vi "Pick and Place Camera.vi"(0 "Gantry In":refnum<k24>, 1 "XYZTheta":dbl[](array[numeric]), 4 "Position":i32, 5 "Tray Number":i32) -> (7 "Gantry Out":refnum<k24>)   [LabVIEW 2021, in "Pick and Place.lvclass"]
uses:
  Pick and Place.lvclass
  Controller/Camera/Image processing.ctl
  Controller/Camera/Camera settings.ctl
  Workspace/Component/Find Component.ctl
  Controller/Camera/Machine Vision.ctl
  C:/Program Files (x86)/Aerotech/A3200/LabVIEW/2010/Bin/Aerotech.A3200.dll
  Program Files (x86)/Aerotech/A3200/LabVIEW/2010/Bin/Aerotech.A3200.dll
  Controller/Camera/Edmund Optics/Edmund Optics.lvclass
  C:/Users/HEP/Documents/GitHub/Gantry/UCSB-Gantry-HEP-main/Classes/Controller/Camera/Camera.lvclass
  Controller/Camera/Camera.lvclass
  Controller/Motion/A3200/A3200.lvclass
  Controller/Motion/Motion.lvclass
  Workspace/Component/Component Tray.lvclass
panel:
  in  "Machine Vision":T1
  in  "Assembly Type":string
  in  "Component":T2
  in  "Verify CH1":bool
  out "CH1 correct?":bool
  in  "Go to Sensor ID":bool
  in  "Go to CH1":bool
  in  "Go to Center":bool
  in  "Joystick":bool
  in  "Focus":bool
  in  "number of focus steps":i32
  in  "Focus step size":dbl format="%#_13g"
  out "XYZTheta 2":dbl[](array[numeric]) format="%.6g"
  out "All fiducials recorded":bool
  out "CH1 Location":dbl[](array[numeric])
  out "Sensor ID Location":dbl[](array[numeric])
  out "XY Graph":cluster{"X":dbl, "Y":dbl}[](graph)
  out "Bottom Left XY":dbl[](array[numeric]) format="%.6g"
  out "Bottom Right XY":dbl[](array[numeric]) format="%.6g"
  out "Top Right XY":dbl[](array[numeric]) format="%.6g"
  out "Top Left XY":dbl[](array[numeric]) format="%.6g"
  in  "Record Top Left":bool
  in  "Record Top Right":bool
  in  "Record Bottom Right":bool
  in  "Record Bottom Left":bool
  in  "Go to Top Left":bool
  in  "Go to Bottom Left":bool
  in  "Go to Bottom Right":bool
  in  "Go to Top Right":bool
  out "Gantry":dbl[](array[numeric]) format="%.6g"
  out "Sum":dbl[](array[numeric]) format="%.6g"
  out "Low Speed":bool
  out "X":bool
  out "Y":bool
  out "Z":bool
  out "High Speed":bool
  in  "Stop Program":bool
  out "Image":T3(plugin-control)
  out "Camera":dbl[](array[numeric]) format="%.6g"
  in  "Override presets":bool
  in  "Camera settings":T4={"Gamma"=1.6, "Gain"=0, "Sharpness"=0, "Contrast"=0.0, "Exposure"=0.0078125} {"Exposure" min=0.000244140625 max=0.5 scale=0.0002..0.5; "Contrast" min=0.0 max=1.0 scale=0.001..1.0; "Sharpness" min=0 max=2 step=1 scale=0.0..2.0; "Gain" min=0 max=100 step=1 scale=0.1..100.0; "Gamma" min=0.01 max=10.0 scale=0.01..10.0}
  in  "Image processing":T5={"Brightness"=128.0, "Contrast"=45.0, "Gamma"=1.0471123} {"Brightness" scale=0.0..400.0; "Contrast" scale=0.0..90.0; "Gamma" scale=0.005..5.0}
  out "Average Strength":dbl
  out "Program Stopped":bool
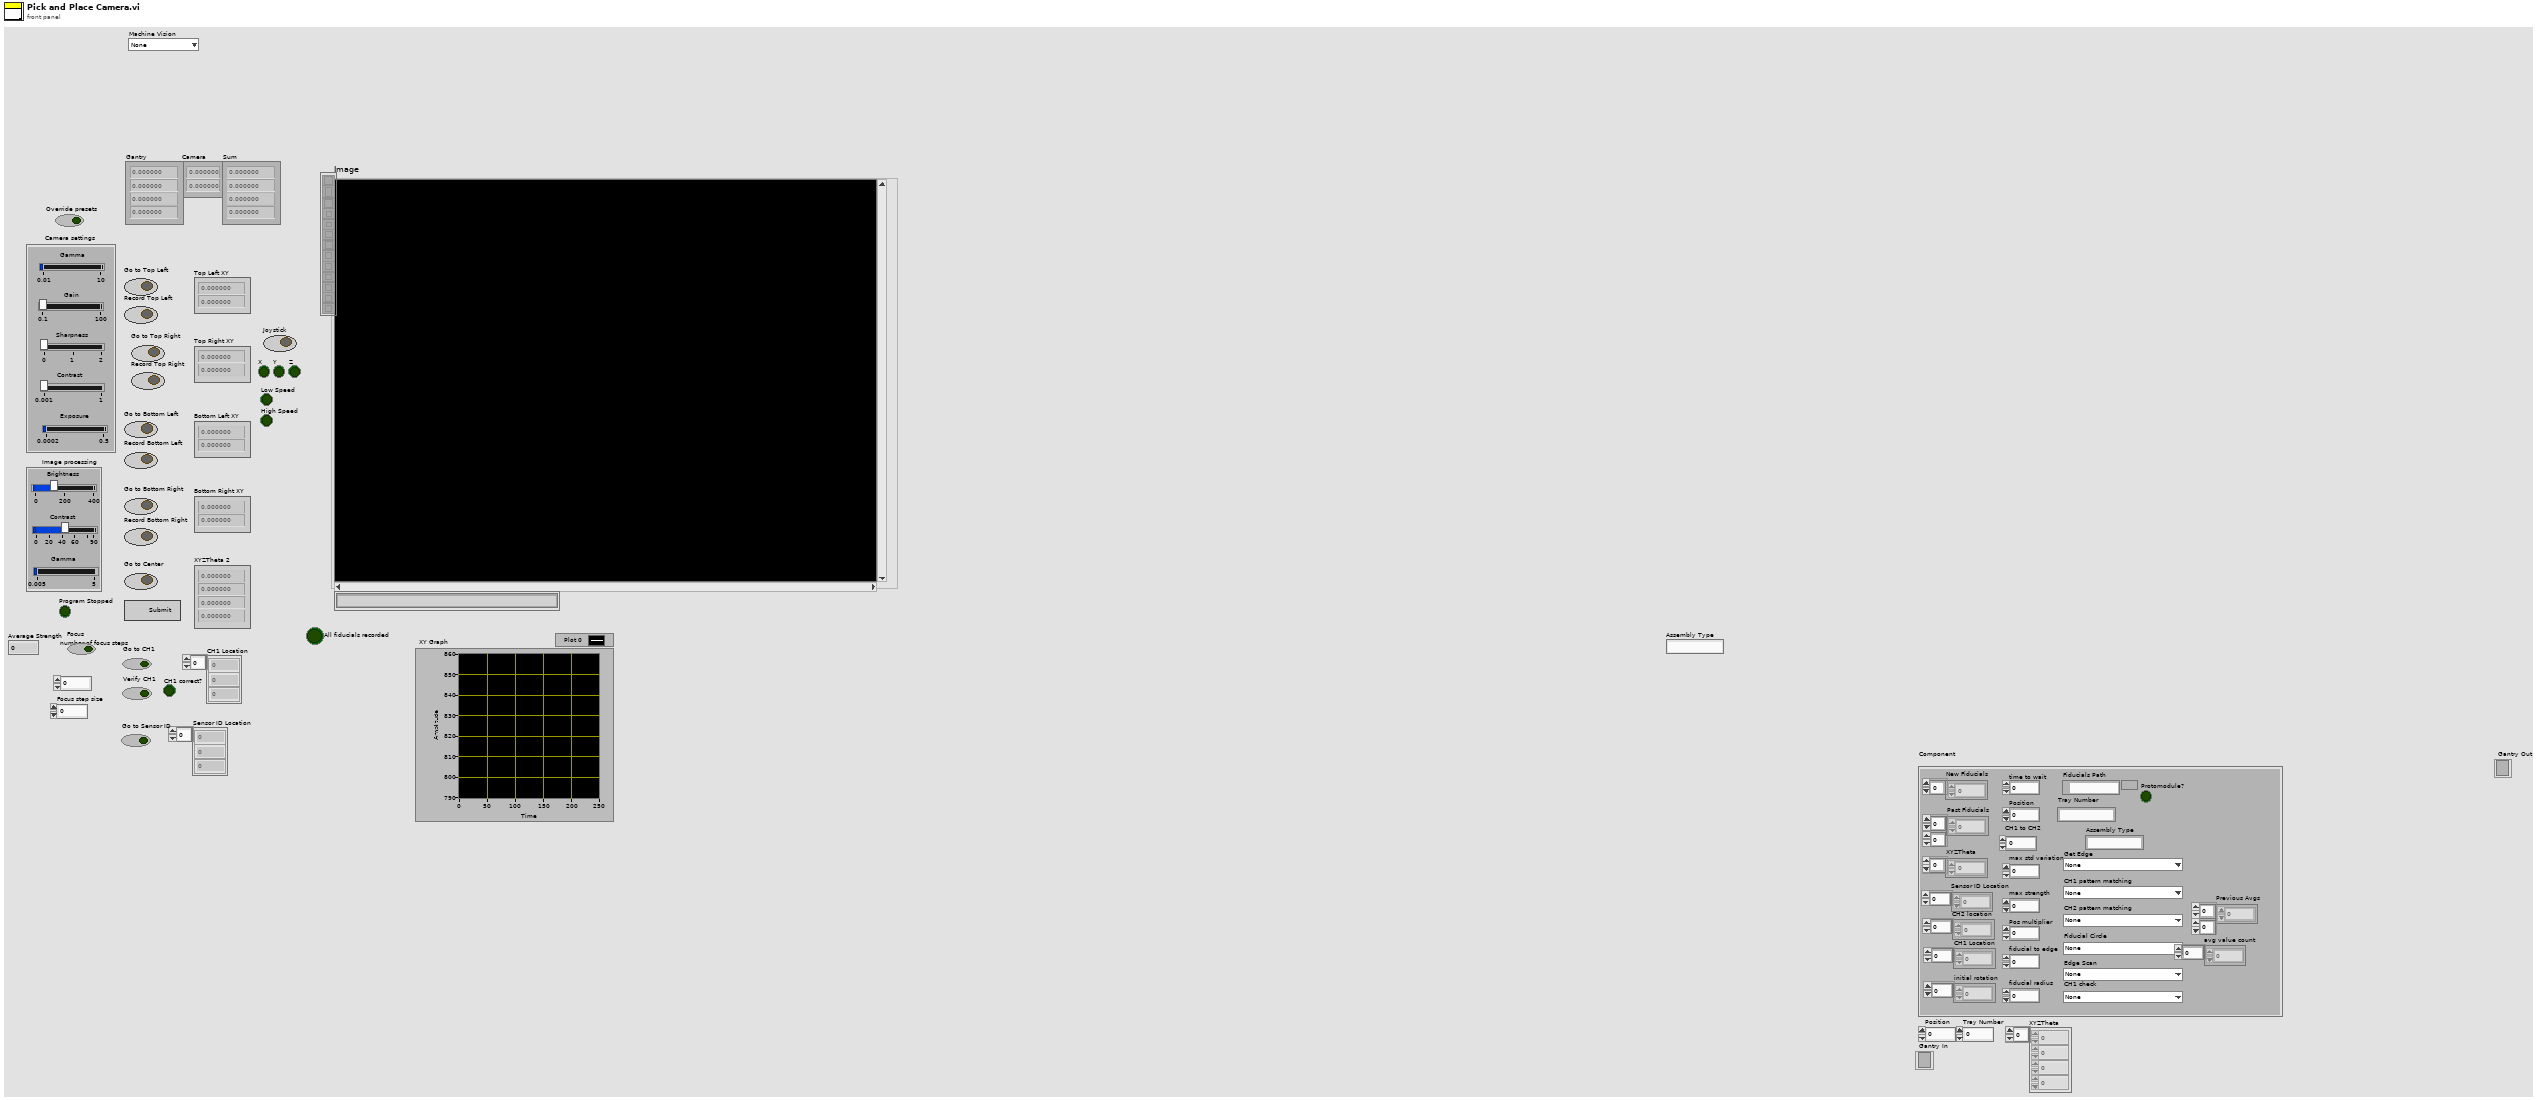
[diagram p1: front panel]
types:
  T1 = typedef "Camera.lvclass/Machine Vision.ctl" = enum16{"None", "Assembly Tray Circle", "Assembly Tray Fiducial", "Partial Hexaboard", "sensor edge init", "HB edge init", "sensor edge pos1", "sensor edge pos2", "HB edge pos1", "HB edge pos2", "Sensor CH1-2", "HB CH1", "HB CH2", "V3 Sensor Circle", "Hexaboard Circle", "sensor CH1 check", "HB CH1 check ", "sensor ID"}
  T2 = typedef "Component Tray.lvclass/Find Component.ctl" = cluster{"New Fiducials":dbl[], "Past Fiducials":dbl[][], "XYZTheta":dbl[], "Fiducials Path":path, "Position":i32, "CH1 Location":dbl[], "Sensor ID Location":dbl[], "initial rotation":dbl[], "CH2 location":dbl[], "max std variation":dbl, "max strength":dbl, "CH2 pattern matching":T1, "Fiducial Circle":T1, "Get Edge":T1, "Pos multiplier":dbl, "time to wait":u32, "fiducial to edge":dbl, "Protomodule?":bool, "Assembly Type":string, "CH1 to CH2":dbl, "Tray Number":string, "fiducial radius":dbl, "4 fiducials?":bool, "CH1 check":T1, "Edge Scan":T1, "CH1 pattern matching":T1, "Sensor Thickness":dbl, "Previous Avgs":dbl[][], "avg value count":dbl[]}
  T3 = typedef "IMAQ Image.ctl" = refnum<image>
  T4 = typedef "Camera.lvclass/Camera settings.ctl" = cluster{"Gamma":dbl, "Gain":i64, "Sharpness":i64, "Contrast":dbl, "Exposure":dbl}
  T5 = typedef "Camera.lvclass/Image processing.ctl" = cluster{"Brightness":sgl, "Contrast":sgl, "Gamma":sgl}
  T6 = cluster{"Average Strength":dbl, "Radius (Real-World)":dbl, "Match found?":bool, "initial angle":sgl, "Global Report":cluster{"Mean Value":sgl, "Standard Variation":sgl, "Minimal Value":sgl, "Maximal Value":sgl, "Area (calibrated)":sgl, "Area (pixels)":u32, "%":sgl, "Calibration Valid":bool}}
  T7 = typedef "File Paths.ctl" = cluster{"Glue Pattern Folder":path, "Carrier Tray Folder":path, "Pick Up Tool Fixture Folder":path, "Components Folder":path, "Bellows Tool Offset.txt":path, "Pick Up Tool Offset.txt":path, "Dispense Tip Offset.txt":path, "Log Files":path, "Gantry Assembly Map.txt":path, "Syringe and offset map.txt":path, "Controllers Folder":path, "Local dbase config":path}
  T8 = enum8{"Enabled", "Disabled", "Disabled and Grayed Out"}
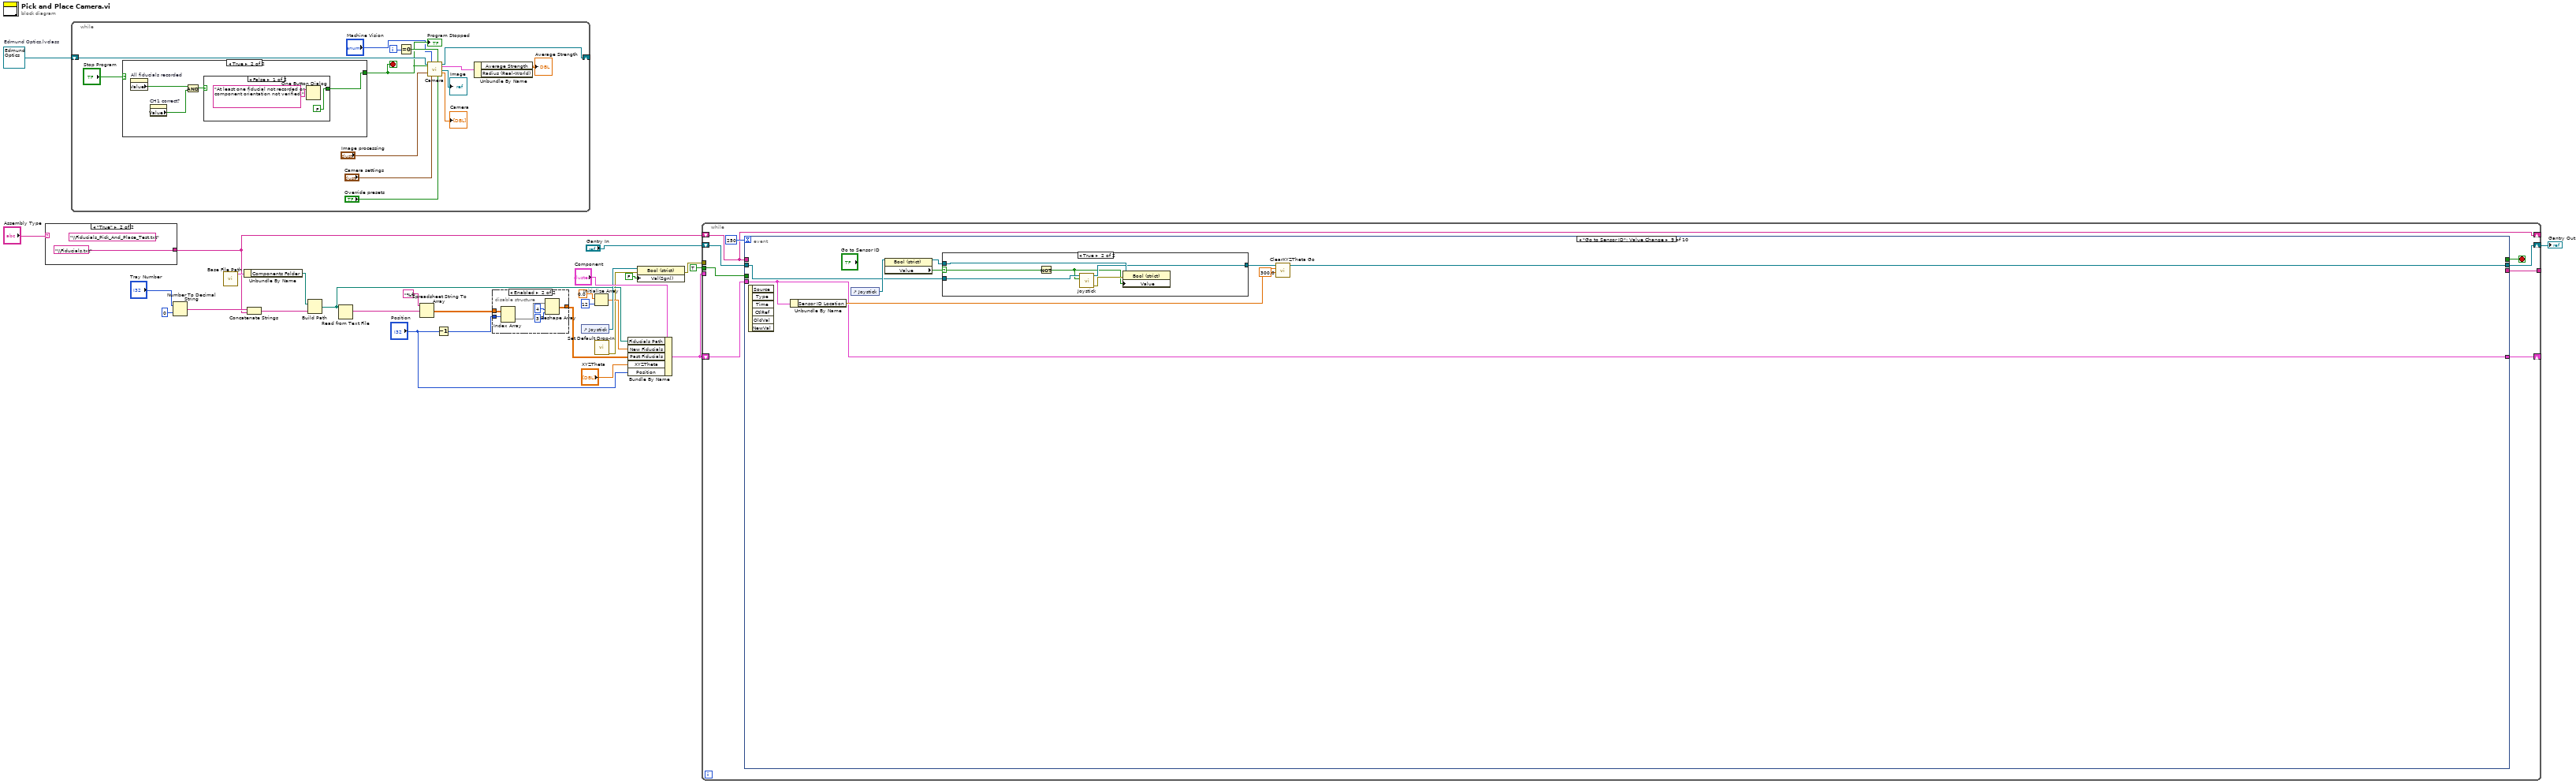
[diagram p0: block diagram]
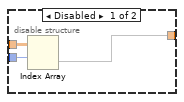
[diagram p2: hidden frame]
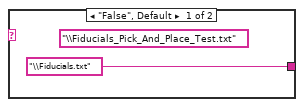
[diagram p3: hidden frame]
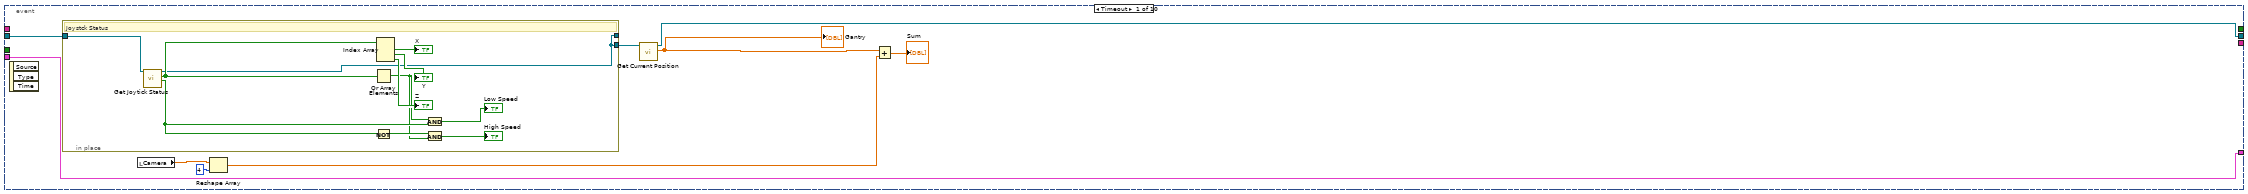
[diagram p4: hidden frame]
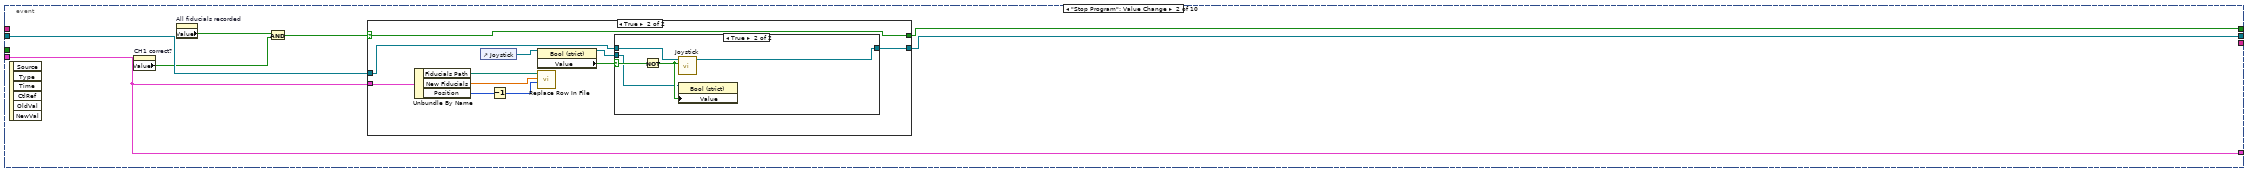
[diagram p5: hidden frame]
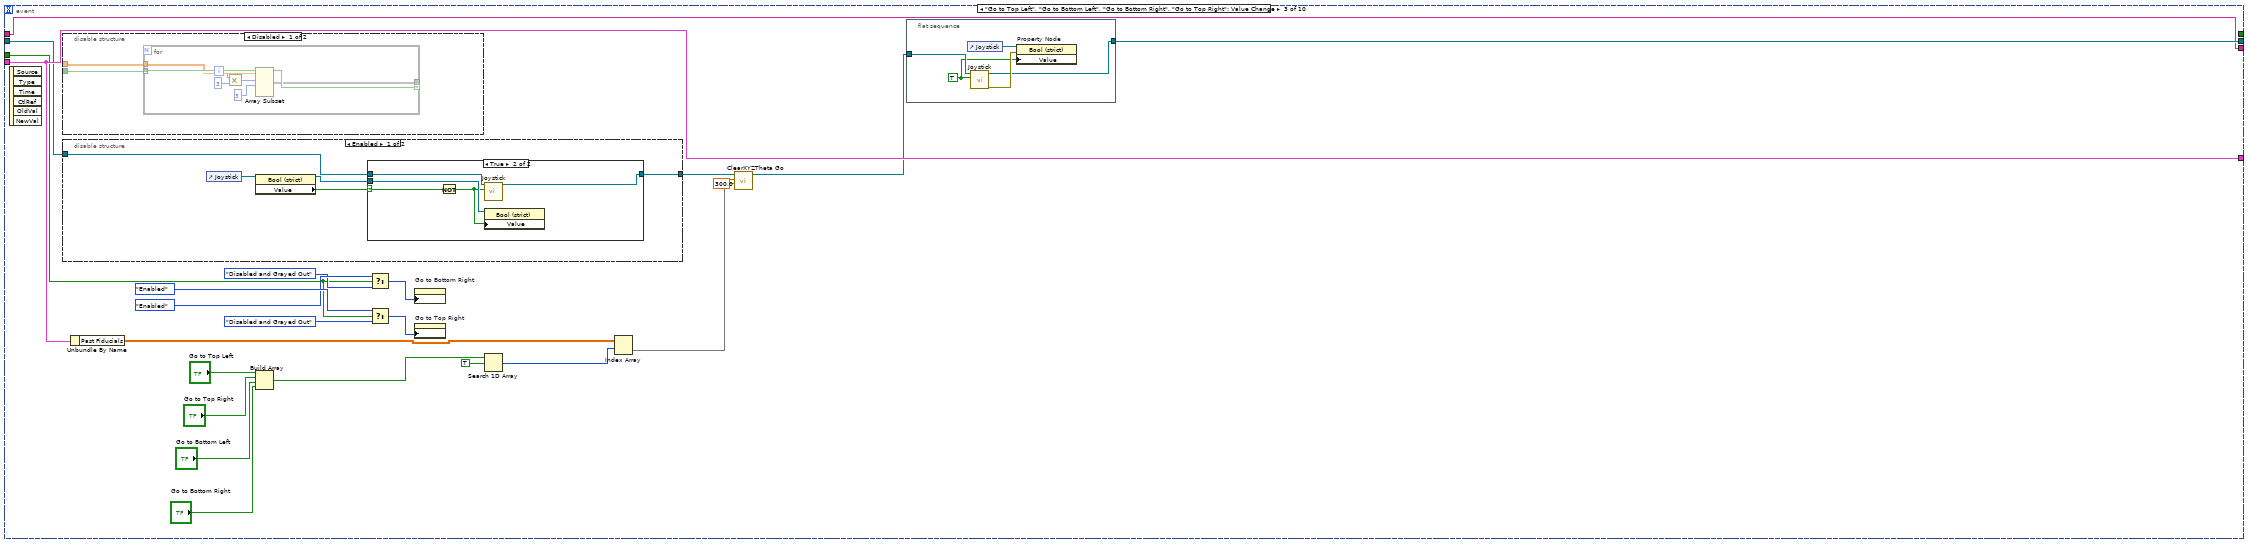
[diagram p8: hidden frame]
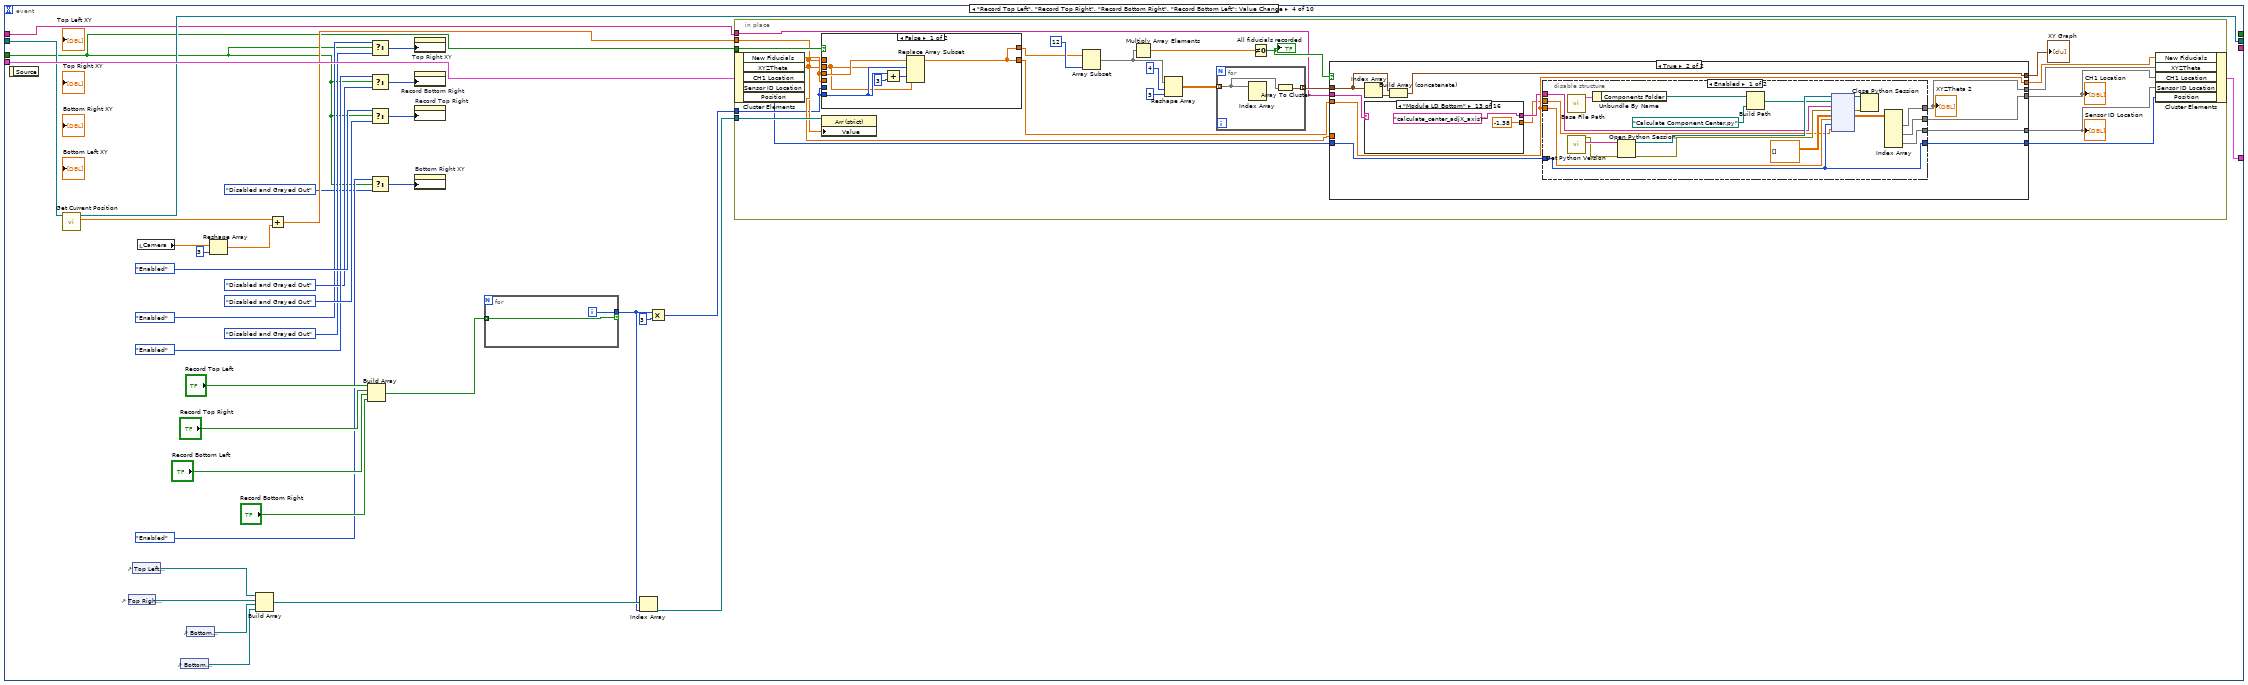
[diagram p12: hidden frame]
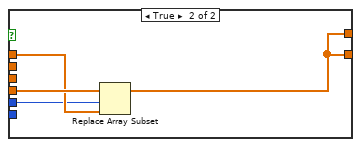
[diagram p13: hidden frame]
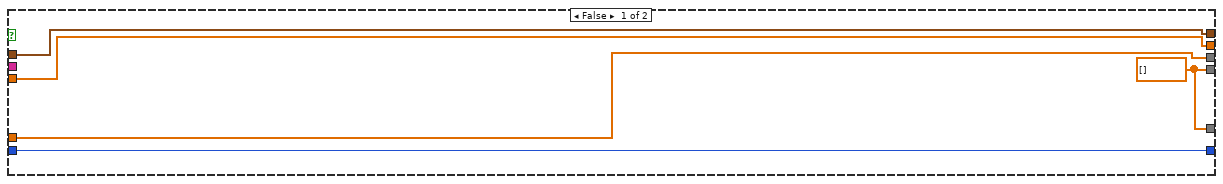
[diagram p14: hidden frame]
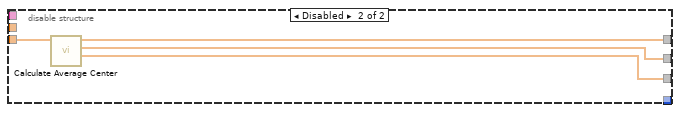
[diagram p15: hidden frame]
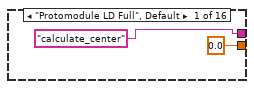
[diagram p16: hidden frame]
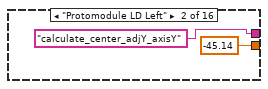
[diagram p17: hidden frame]
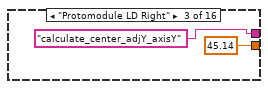
[diagram p18: hidden frame]
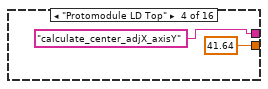
[diagram p19: hidden frame]
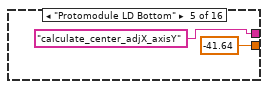
[diagram p20: hidden frame]
diagram:
  w25 = refnum<class "Edmund Optics.lvclass"> refnum  # Edmund Optics.lvclass
  n1 = case shown="\"True\"" "Assembly Type" {
    tunnel: ["\\Fiducials.txt" ("string") "\\Fiducials.txt" ("string")] -> w3
    frame "False", Default {
      (unwired) "\\Fiducials_Pick_And_Place_Test.txt" ("string")
    }
    frame "True" {
      (unwired) "\\Fiducials_Pick_And_Place_Test.txt" ("string")
    }
  }
  n2 = while {
    shift-right: [w42] -> _
    shift-left: w25 -> [w45]
    i -> [w38]
    stop <- w35 stop-if-true
    n3 = case shown="True" "Stop Program" {
      tunnel: [FALSE w47] -> w35
      frame False {
      }
      frame True {
        n4 = property on="All fiducials recorded" class="Bool (strict)"() -> ("Value"=w50:bool)  [unwired: 2 in, 2 out]
        n5 = property on="CH1 correct?" class="Bool (strict)"() -> ("Value"=w48:bool)  [unwired: 2 in, 2 out]
        n6 = And(x=w50, y=w48) -> (x .and. y?=w49:bool)
        n7 = case shown="False" w49 {
          tunnel: [FALSE TRUE] -> w47
          frame False {
            n8 = One Button Dialog(message="At least one fiducial not recorded or component orientation not verified.") -> ()  [unwired: 1 in, 1 out]
          }
          frame True {
            n9 = property on="All fiducials recorded" class="Bool (strict)"("Val(Sgnl)"=FALSE) -> ()  [unwired: 2 in, 2 out]
          }
        }
      }
    }
    "Program Stopped" <- w35
    n10 = Equal To 0?(x=w38) -> (x = 0?=w37:bool)
    n11 = call "Camera.vi"("Camera in"=w45, "Stop"=w35, "BCG Image Processing"="Image processing", "Machine Vision"="Machine Vision", "Camera settings"="Camera settings", "Loop 0"=w37, "Override presets"="Override presets") -> ("Camera out"=w42:refnum<class "Edmund Optics.lvclass">, "output cluster"=w33:T6, "Image"=→"Image":T3, "Camera"=→"Camera":dbl[])  [unwired: 5 in, 4 out]
    n12 = Unbundle By Name(w33) -> ("Average Strength"=→"Average Strength":dbl)  [unwired: 1 out]
  }
  n13 = Number To Decimal String(number="Tray Number", width (-)=i16 0) -> (decimal integer string=w20:string)
  n14 = call "Base File Path.vi"() -> ("Paths Out"=w17:T7)  [unwired: 11 in]
  n15 = Unbundle By Name(w17) -> ("Components Folder"=w19:path)
  n16 = Concatenate Strings "Concatenate Strings"(w20, w3) -> (w21:string)
  n17 = Build Path(base path=w19, name or relative path=w21) -> (appended path=w12:path)
  n18 = Read from Text File(file (use dialog)=w12) -> (text=w22:string)  [unwired: 3 in, 3 out]
  n19 = Spreadsheet String To Array(format string="%f", spreadsheet string=w22) -> (array=w24:dbl[][])  [unwired: 2 in]
  n20 = Decrement(x="Position") -> (x-1=w9:i32)
  n21 = disable-structure shown="Enabled" {
    disable-tunnel: w24 -> [w57 w59]
    disable-tunnel: w9 -> [w56 w60]
    disable-tunnel: [w55 w58] -> w2
    frame Disabled {
      n22 = Index Array "Index Array"(array=w57, index (row)=w56) -> (element=w55:dbl[])  [unwired: 1 in]
    }
    frame Enabled {
      n23 = Index Array "Index Array"(array=w59, index (row)=w60) -> (element=w63:dbl[])  [unwired: 1 in]
      n24 = Reshape Array(w63, 4 ("dimension size"), 3 ("dimension size")) -> (w58:dbl[][])
    }
  }
  n25 = control-ref of="Joystick"() -> (w28:refnum<vi>)
  n26 = Initialize Array(0.0 ("element"), 12 ("dimension size")) -> (w15:dbl[])
  n27 = call "Set Default Drop-In.vi"() -> ("error out"=w8:errorcluster)  [unwired: 11 in]
  n28 = Bundle By Name "Bundle By Name"(cluster="Component", "Fiducials Path"=w12, "New Fiducials"=w15, "Past Fiducials"=w2, "XYZTheta"="XYZTheta", "Position"="Position") -> (w6:T2)
  n29 = property class="Bool (strict)"(reference=w28, error in=w8, "Val(Sgnl)"=FALSE) -> (error out=w26:errorcluster)  [unwired: 1 out]
  n30 = while {
    shift-right: [w70] -> _
    shift-left: w6 -> [w71]
    tunnel: w26 -> [_]
    shift-right: [w67] -> w7
    shift-left: "Gantry In" -> [w68]
    tunnel: w6 -> [_]
    tunnel: [w66] -> _
    tunnel: TRUE -> [w65]
    shift-right: [w64] -> _
    shift-left: w3 -> [w64]
    stop <- w72 stop-if-true
    n31 = event shown="[8] \"Go to Sensor ID\": Value Change" {
      selector: _ -> [_ _ _ _ _ _ _ _ _ _]
      dyn-events: _ -> [_ _ _ _ _ _ _ _ _ _]
      timeout: 250 -> [_ _ _ _ _ _ _ _ _ _]
      tunnel: [_ w96 _ _ _ _ _ _ _ _] -> w72
      tunnel: w71 -> [w80 w98 w141 w203 w323 w369 w377 w393 w409 w419]
      tunnel: [w80 w98 w141 w202 w323 w369 w377 w393 w409 w419] -> w70
      tunnel: w68 -> [w74 w99 w140 w194 w325 w368 w373 w389 w405 w420]
      tunnel: [w76 w97 w137 w192 w324 w366 w371 w387 w403 w420] -> w67
      tunnel: w64 -> [_ _ w134 w191 _ _ _ _ _ _]
      tunnel: [_ _ w134 _ _ _ _ _ _ _] -> w66
      tunnel: w65 -> [_ _ w125 w167 _ _ _ _ _ _]
      event Timeout {
        n32 = event-data() -> ()  [unwired: 1 in, 3 out]
        n33 = in-place {
          in-place-border: w74 -> [w92]
          in-place-border: [w82] -> _
          in-place-border: [w82] -> w73
          # "Joystck Status"
          n34 = call "Get Joytick Status.vi"("Gantry In"=w92) -> ("JoystickLowSpeedActive"=w86:bool, "Joystick Status"=w88:bool[], "Gantry Out"=w82:refnum<k24>)  [unwired: 5 in, 3 out]
          n35 = Or Array Elements(Boolean array=w88) -> (logical OR=w84:bool)
          n36 = Not(x=w86) -> (.not. x?=w85:bool)
          n37 = Index Array(array=w88) -> (element #1=→"X":bool, element #2=→"Y":bool, element #3=→"Z":bool)  [unwired: 3 in]
          n38 = And(x=w84, y=w86) -> (x .and. y?=→"Low Speed":bool)
          n39 = And(x=w85, y=w84) -> (x .and. y?=→"High Speed":bool)
        }
        n40 = local read "Camera"() -> (w79:dbl[])
        n41 = Reshape Array(w79, 4 ("dimension size")) -> (w77:dbl[])
        n42 = call "Get Current Position.vi"("Gantry In"=w73) -> ("XYZTheta Out"=w75:dbl[], "Gantry Out"=w76:refnum<k24>)  [unwired: 8 in, 1 out]
        "Gantry" <- w75
        n43 = Add(x=w75, y=w77) -> (x+y=→"Sum":dbl[])
      }
      event "Stop Program": Value Change {
        n44 = event-data() -> ()  [unwired: 1 in, 6 out]
        n45 = property on="CH1 correct?" class="Bool (strict)"() -> ("Value"=w95:bool)  [unwired: 2 in, 2 out]
        n46 = property on="All fiducials recorded" class="Bool (strict)"() -> ("Value"=w94:bool)  [unwired: 2 in, 2 out]
        n47 = And(x=w94, y=w95) -> (x .and. y?=w93:bool)
        n48 = case shown="True" w93 {
          selector: w93 -> [w100 w109]
          tunnel: w99 -> [w101 w111]
          tunnel: w98 -> [_ w112]
          tunnel: [w101 w110] -> w97
          tunnel: [w100 w109] -> w96
          frame False {
          }
          frame True {
            n49 = Unbundle By Name(w112) -> ("Fiducials Path"=w106:path, "New Fiducials"=w105:dbl[], "Position"=w107:i32)
            n50 = control-ref of="Joystick"() -> (w103:refnum<vi>)
            n51 = Decrement(x=w107) -> (x-1=w108:i32)
            n52 = property class="Bool (strict)"(reference=w103) -> (reference out=w102:refnum<vi>, "Value"=w104:bool)  [unwired: 1 in, 1 out]
            n53 = call "Replace Row In File.vi"("Index"=w108, "Insert Array"=w105, "Path"=w106) -> ()  [unwired: 8 in, 1 out]
            n54 = case shown="True" w104 {
              selector: w104 -> [_ w118]
              tunnel: w111 -> [w113 w117]
              tunnel: [w113 w116] -> w110
              tunnel: w102 -> [_ w114]
              frame False {
              }
              frame True {
                n55 = Not(x=w118) -> (.not. x?=w115:bool)
                n56 = call "Joystick.vi"("Joystick"=w115, "Gantry In"=w117) -> ("Gantry Out"=w116:refnum<k24>)  [unwired: 8 in, 1 out]
                n57 = property class="Bool (strict)"(reference=w114, "Value"=w115) -> ()  [unwired: 1 in, 2 out]
              }
            }
          }
        }
      }
      event "Go to Top Left", "Go to Bottom Left", "Go to Bottom Right", "Go to Top Right": Value Change {
        n58 = event-data() -> ()  [unwired: 1 in, 6 out]
        n59 = disable-structure shown="Disabled" {
          disable-tunnel: _ -> [w143 _]
          disable-tunnel: _ -> [w142 _]
          frame Disabled {
            n60 = for {
              tunnel: w143 -> [w150] mode=indexing
              tunnel: w142 -> [w149]
              tunnel: [w144] -> _ if=w150
              i -> [w147]
              n61 = Multiply(x=w147, y=3) -> (x*y=w145:i32)
              n62 = Array Subset "Array Subset"(array=w149, index (row)=w145, length (row)=3 ("length")) -> (w144:void[][])  [unwired: 2 in]
            }
          }
          frame Enabled {
          }
        }
        n63 = disable-structure shown="Enabled" {
          disable-tunnel: w140 -> [w153 _]
          disable-tunnel: [w152 _] -> w139
          frame Enabled {
            n64 = control-ref of="Joystick"() -> (w151:refnum<vi>)
            n65 = property class="Bool (strict)"(reference=w151) -> (reference out=w154:refnum<vi>, "Value"=w155:bool)  [unwired: 1 in, 1 out]
            n66 = case shown="True" w155 {
              selector: w155 -> [_ w161]
              tunnel: w153 -> [w156 w159]
              tunnel: [w156 w157] -> w152
              tunnel: w154 -> [_ w160]
              frame False {
              }
              frame True {
                n67 = Not(x=w161) -> (.not. x?=w158:bool)
                n68 = call "Joystick.vi"("Joystick"=w158, "Gantry In"=w159) -> ("Gantry Out"=w157:refnum<k24>)  [unwired: 8 in, 1 out]
                n69 = property class="Bool (strict)"(reference=w160, "Value"=w158) -> ()  [unwired: 1 in, 2 out]
              }
            }
          }
          frame Disabled {
          }
        }
        n70 = Unbundle By Name(w141) -> ("Past Fiducials"=w122:dbl[][])
        n71 = Build Array "Build Array"("Go to Top Left", "Go to Top Right", "Go to Bottom Left", "Go to Bottom Right") -> (w121:bool[])
        n72 = Select(t=T8."Enabled" ("Disabled"), s=w125, f=T8."Disabled and Grayed Out" ("Disabled")) -> (s? t:f=w126:T8)
        n73 = Select(t=T8."Enabled" ("Disabled"), s=w125, f=T8."Disabled and Grayed Out" ("Disabled")) -> (s? t:f=w129:T8)
        n74 = property on="Go to Bottom Right" class="Bool"("DisabledEnum"=w126) -> ()  [unwired: 2 in, 2 out]
        n75 = property on="Go to Top Right" class="Bool"("DisabledEnum"=w129) -> ()  [unwired: 2 in, 2 out]
        n76 = Search 1D Array(1D array=w121, element=TRUE) -> (index of element=w123:i32)  [unwired: 1 in]
        n77 = Index Array(array=w122, index (row)=w123) -> (element=w120:dbl[])  [unwired: 1 in]
        n78 = call "ClearXYZTheta Go.vi"("Speed"=300.0, "XYZTheta In"=w120, "Gantry In"=w139) -> ("Gantry Out"=w138:refnum<k24>)  [unwired: 6 in, 2 out]
        n79 = flat-sequence {
          tunnel: w138 -> [w166]
          tunnel: [w163] -> w137
          frame #0 {
            w162 = TRUE
            n80 = control-ref of="Joystick"() -> (w165:refnum<vi>)
            n81 = call "Joystick.vi"("Joystick"=w162, "Gantry In"=w166) -> ("error out"=w164:errorcluster, "Gantry Out"=w163:refnum<k24>)  [unwired: 8 in]
            n82 = property on="Property Node" class="Bool (strict)"(reference=w165, error in=w164, "Value"=w162) -> ()  [unwired: 2 out]
          }
        }
      }
      event "Record Top Left", "Record Top Right", "Record Bottom Right", "Record Bottom Left": Value Change {
        n83 = event-data() -> ()  [unwired: 1 in, 1 out]
        n84 = call "Get Current Position.vi"("Gantry In"=w194) -> ("XYZTheta Out"=w193:dbl[], "Gantry Out"=w192:refnum<k24>)  [unwired: 8 in, 1 out]
        n85 = control-ref of="Top Right XY"() -> (w188:refnum<vi>)
        n86 = control-ref of="Top Left XY"() -> (w189:refnum<vi>)
        n87 = local read "Camera"() -> (w197:dbl[])
        n88 = control-ref of="Bottom Right XY"() -> (w186:refnum<vi>)
        n89 = control-ref of="Bottom Left XY"() -> (w187:refnum<vi>)
        n90 = Reshape Array(w197, 3 ("dimension size")) -> (w196:dbl[])
        n91 = Build Array "Build Array"(w189, w188, w187, w186) -> (w201:refnum<vi>[])
        n92 = Add(x=w193, y=w196) -> (x+y=w195:dbl[])
        n93 = Build Array "Build Array"("Record Top Left", "Record Top Right", "Record Bottom Left", "Record Bottom Right") -> (w190:bool[])
        n94 = Select(t=T8."Enabled" ("Disabled"), s=w167, f=T8."Disabled and Grayed Out" ("Disabled")) -> (s? t:f=w172:T8)
        n95 = Select(t=T8."Enabled" ("Disabled"), s=w167, f=T8."Disabled and Grayed Out") -> (s? t:f=w176:T8)
        n96 = Select(t=T8."Enabled" ("Disabled"), s=w167, f=T8."Disabled and Grayed Out") -> (s? t:f=w178:T8)
        n97 = Select(t=T8."Enabled" ("Disabled"), s=w167, f=T8."Disabled and Grayed Out" ("Disabled")) -> (s? t:f=w168:T8)
        n98 = property on="Top Right XY" class="Arr (strict)"("DisabledEnum"=w172) -> ()  [unwired: 2 in, 2 out]
        n99 = property on="Record Bottom Right" class="Bool"("DisabledEnum"=w176) -> ()  [unwired: 2 in, 2 out]
        n100 = property on="Record Top Right" class="Bool"("DisabledEnum"=w178) -> ()  [unwired: 2 in, 2 out]
        n101 = property on="Bottom Right XY" class="Arr (strict)"("DisabledEnum"=w168) -> ()  [unwired: 2 in, 2 out]
        n102 = for {
          tunnel: w190 -> [w204] mode=indexing
          tunnel: [w205] -> w181 if=w204
          i -> [w205]
        }
        n103 = Index Array "Index Array"(array=w201, index=w181) -> (element=w200:refnum<vi>)
        n104 = Multiply(x=w181, y=3) -> (x*y=w198:i32)
        n105 = in-place {
          in-place-border: w198 -> [w209]
          in-place-border: w200 -> [w227]
          in-place-border: w195 -> [w210]
          in-place-border: w191 -> [w214]
          in-place-border: w167 -> [w212]
          n106 = in-place-cluster #1(w203) -> ("New Fiducials"=w211:dbl[], "XYZTheta"=w226:dbl[], "Position"=w207:i32)  [unwired: 2 out]
          n107 = case shown="False" w212 {
            tunnel: w211 -> [w235 _]
            tunnel: w209 -> [w234 _]
            tunnel: w210 -> [w233 _]
            tunnel: [w230 w236] -> w213
            tunnel: w211 -> [_ w239]
            tunnel: w210 -> [_ w238]
            tunnel: w209 -> [_ w237]
            tunnel: [w230 w236] -> w208
            frame False {
              n108 = Add(x=w234, y=3) -> (x+y=w231:i32)
              n109 = Replace Array Subset "Replace Array Subset"(array=w235, new element #1=w233, index #1=w234, new element #2=w233, index #2=w231) -> (w230:dbl[])
            }
            frame True {
              n110 = Replace Array Subset "Replace Array Subset"(array=w239, new element=w238, index=w237) -> (w236:dbl[])
            }
          }
          n111 = property class="Arr (strict)"(reference=w227, "Value"=w210) -> ()  [unwired: 1 in, 2 out]
          n112 = Array Subset "Array Subset"(array=w208, length=12) -> (w221:dbl[])  [unwired: 1 in]
          n113 = Multiply Array Elements(1:w221) -> (0:w224:dbl)
          n114 = Reshape Array "Reshape Array"(w221, 4 ("dimension size"), 3 ("dimension size")) -> (w218:dbl[][])
          n115 = for {
            tunnel: w218 -> [w240] mode=indexing
            tunnel: [w241] -> w217 mode=indexing
            n116 = Index Array(array=w240) -> ()  [unwired: 2 in, 2 out]
            n117 = Array To Cluster(array=w240) -> (cluster=w241:cluster{"[0]":dbl, "[1]":dbl})
          }
          n118 = Not Equal To 0?(x=w224) -> (x != 0?=w215:bool)
          "All fiducials recorded" <- w215
          n119 = case shown="True" w215 {
            tunnel: [w245 w251] -> w229
            tunnel: w213 -> [w246 w255]
            tunnel: [w246 w255] -> w228
            tunnel: w226 -> [w245 _]
            tunnel: [w244 w252] -> w223
            tunnel: [w244 w253] -> w222
            tunnel: w217 -> [w243 w258]
            tunnel: [w243 w256] -> w216
            tunnel: w214 -> [_ w254]
            tunnel: w207 -> [w242 w249]
            tunnel: [w242 w248] -> w206
            frame False {
              w244 = dbl[] [] ("CH1 location")
            }
            frame True {
              n120 = Index Array(array=w258) -> (element=w257:cluster{"[0]":dbl, "[1]":dbl})  [unwired: 1 in]
              n121 = case shown="\"Module LD Bottom\"" w254 {
                tunnel: ["calculate_center" ("function name") "calculate_center_adjY_axisY" ("function name") "calculate_center_adjY_axisY" ("function name") "calculate_center_adjX_axisY" ("function name") "calculate_center_adjX_axisY" ("function name") "calculate_center" ("function name") "calculate_center" ("function name") "calculate_center_adjX_axisY" ("function name") "calculate_center" ("function name") "calculate_center_adjY_axisX" ("function name") "calculate_center_adjY_axisX" ("function name") "calculate_center_adjX_axisY" ("function name") "calculate_center_adjX_axisY" ("function name") "calculate_center_adjY_axisX" ("function name") "calculate_center" ("function name") "calculate_center_adjX_axisY" ("function name")] -> w250
                tunnel: [0.0 -45.14 45.14 41.64 -41.64 0.0 0.0 49.78 0.0 -2.0 13.0 2.0 -1.38 0.0 0.0 21.0] -> w247
                frame "Protomodule LD Full", Default {
                }
                frame "Protomodule LD Left" {
                }
                frame "Protomodule LD Right" {
                }
                frame "Protomodule LD Top" {
                }
                frame "Protomodule LD Bottom" {
                }
                frame "Protomodule LD Five" {
                }
                frame "Protomodule HD Full" {
                }
                frame "Protomodule HD Top" {
                }
                frame "Module LD Full" {
                }
                frame "Module LD Left" {
                }
                frame "Module LD Right" {
                }
                frame "Module LD Top" {
                }
                frame "Module LD Bottom" {
                }
                frame "Module LD Five" {
                }
                frame "Module HD Full" {
                }
                frame "Module HD Top" {
                }
              }
              n122 = Build Array (concatenate)(w258, w257) -> (w256:cluster{"[0]":dbl, "[1]":dbl}[])
              n123 = disable-structure shown="Enabled" {
                disable-tunnel: w255 -> [w268 w278]
                disable-tunnel: [w264 w281] -> w253
                disable-tunnel: [w265 w280] -> w252
                disable-tunnel: [w266 w279] -> w251
                disable-tunnel: w250 -> [w263 _]
                disable-tunnel: w249 -> [w260 _]
                disable-tunnel: [w260 _] -> w248
                disable-tunnel: w247 -> [w259 _]
                frame Enabled {
                  n124 = call "Base File Path.vi"() -> ("Paths Out"=w273:T7)  [unwired: 11 in]
                  n125 = call "Get Python Version.vi"() -> ("Python Version"=w262:string, "error out"=w261:errorcluster)  [unwired: 10 in]
                  n126 = Unbundle By Name(w273) -> ("Components Folder"=w271:path)
                  n127 = Open Python Session(python version=w262, 3:w261) -> (session out=w277:refnum<k35>, error out=w275:errorcluster)  [unwired: 1 in]
                  n128 = Build Path(base path=w271, name or relative path=path "Calculate Component Center.py") -> (appended path=w270:path)
                  n129 = node(w277, w270, w263, w275, dbl[][] [], w268, w260, w259) -> (w276:refnum<k35>, w274:errorcluster, w267:dbl[][])  [unwired: 3 in, 2 out]
                  n130 = Close Python Session(session in=w276, error in=w274) -> ()  [unwired: 1 out]
                  n131 = Index Array(array=w267) -> (element #1=w266:dbl[], element #2=w265:dbl[], element #3=w264:dbl[])  [unwired: 6 in]
                }
                frame Disabled {
                  n132 = call "Calculate Average Center.vi"("Gantry Fiducials"=w278) -> ("Sensor ID Location"=w281:dbl[], "CH1 Location"=w280:dbl[], "XYZTheta"=w279:dbl[])  [unwired: 8 in]
                }
              }
              "XYZTheta 2" <- w251
            }
          }
          "CH1 Location" <- w223
          "Sensor ID Location" <- w222
          "XY Graph" <- w216
          n133 = in-place-cluster #1("New Fiducials"=w228, "XYZTheta"=w229, "CH1 Location"=w223, "Sensor ID Location"=w222, "Position"=w206) -> (w202:T2)
        }
      }
      event "Focus": Value Change {
        n134 = event-data() -> ()  [unwired: 1 in, 6 out]
        n135 = Divide(x="number of focus steps", y=2) -> (x/y=w328:dbl)
        n136 = Multiply(x=w328, y="Focus step size") -> (x*y=w326:dbl)
        n137 = call "Joystick.vi"("Joystick"=FALSE, "Gantry In"=w325) -> ("Gantry Out"=w319:refnum<k24>)  [unwired: 8 in, 1 out]
        n138 = Negate(x=w326) -> (-x=w320:dbl)
        n139 = call "Z Go.vi"("Increment"=TRUE, "Return Immediately"=FALSE ("Increment"), "Speed In"=1.0 ("Speed"), "Position In"=w320, "Gantry In"=w319) -> ("error out"=w317:errorcluster, "Gantry Out"=w318:refnum<k24>)  [unwired: 3 in, 2 out]
        n140 = for {
          N: "number of focus steps" -> [_]
          tunnel: [w345] -> w339 mode=indexing
          tunnel: w317 -> [w344]
          tunnel: [w342] -> w332
          shift-right: [w346] -> w333
          shift-left: w318 -> [w348]
          tunnel: "Focus step size" -> [w341]
          n141 = flat-sequence {
            tunnel: w348 -> [w356]
            tunnel: [w355] -> w347
            tunnel: w344 -> [w354]
            tunnel: [w353] -> w343
            tunnel: w341 -> [w351]
            tunnel: w347 -> [w365]
            tunnel: [w364] -> w346
            tunnel: [w363] -> w345
            tunnel: w343 -> [w359]
            tunnel: [w358] -> w342
            frame #0 {
              n142 = call "Z Go.vi"("Increment"=TRUE, "Return Immediately"=FALSE ("Increment"), "error in (no error)"=w354, "Speed In"=0.1 ("Speed"), "Position In"=w351, "Gantry In"=w356) -> ("error out"=w353:errorcluster, "Gantry Out"=w355:refnum<k24>)  [unwired: 2 in, 2 out]
            }
            frame #1 {
              n143 = call "Get Current Position.vi"("error in (no error)"=w359, "Gantry In"=w365) -> ("error out"=w358:errorcluster, "XYZTheta Out"=w362:dbl[], "Gantry Out"=w364:refnum<k24>)  [unwired: 7 in]
              n144 = local read "Average Strength"() -> (w357:dbl)
              n145 = Delete From Array(array=w362, index=2) -> (deleted portion=w360:dbl)  [unwired: 1 in, 1 out]
              n146 = Build Array(w357, w360) -> (w363:dbl[])
            }
          }
        }
        n147 = Transpose 2D Array(2D array=w339) -> (transposed array=w338:dbl[][])
        n148 = Index Array(array=w338) -> (element #2=w337:dbl[])  [unwired: 4 in, 1 out]
        n149 = Index Array(array=w338) -> (element=w340:dbl[])  [unwired: 2 in]
        n150 = Array Max & Min(array=w340) -> (max index (indices)=w336:i32)  [unwired: 3 out]
        n151 = Index Array(array=w337, index=w336) -> (element=w335:dbl)
        n152 = call "Z Go.vi"("Increment"=FALSE, "Return Immediately"=FALSE ("Increment"), "error in (no error)"=w332, "Speed In"=15.0 ("Speed"), "Position In"=w335, "Gantry In"=w333) -> ("Gantry Out"=w324:refnum<k24>)  [unwired: 2 in, 3 out]
      }
      event "Joystick": Value Change {
        n153 = event-data() -> ()  [unwired: 1 in, 6 out]
        n154 = call "Joystick.vi"("Joystick"="Joystick", "Gantry In"=w368) -> ("Gantry Out"=w366:refnum<k24>)  [unwired: 8 in, 1 out]
      }
      event "Go to Center": Value Change {
        n155 = event-data() -> ()  [unwired: 1 in, 6 out]
        n156 = Unbundle By Name(w377) -> ("XYZTheta"=w378:dbl[])
        n157 = control-ref of="Joystick"() -> (w374:refnum<vi>)
        n158 = property class="Bool (strict)"(reference=w374) -> (reference out=w375:refnum<vi>, "Value"=w376:bool)  [unwired: 1 in, 1 out]
        n159 = case shown="True" w376 {
          selector: w376 -> [_ w385]
          tunnel: w373 -> [w379 w382]
          tunnel: [w379 w381] -> w372
          tunnel: w375 -> [_ w384]
          frame False {
          }
          frame True {
            n160 = Not(x=w385) -> (.not. x?=w380:bool)
            n161 = call "Joystick.vi"("Joystick"=w380, "Gantry In"=w382) -> ("error out"=w383:errorcluster, "Gantry Out"=w381:refnum<k24>)  [unwired: 8 in]
            n162 = property class="Bool (strict)"(reference=w384, error in=w383, "Value"=w380) -> ()  [unwired: 2 out]
          }
        }
        n163 = call "ClearXYZTheta Go.vi"("Speed"=300.0, "XYZTheta In"=w378, "Gantry In"=w372) -> ("Gantry Out"=w371:refnum<k24>)  [unwired: 6 in, 2 out]
      }
      event "Go to CH1": Value Change {
        n164 = event-data() -> ()  [unwired: 1 in, 6 out]
        n165 = Unbundle By Name(w393) -> ("CH1 Location"=w394:dbl[])
        n166 = control-ref of="Joystick"() -> (w390:refnum<vi>)
        n167 = property class="Bool (strict)"(reference=w390) -> (reference out=w391:refnum<vi>, "Value"=w392:bool)  [unwired: 1 in, 1 out]
        n168 = case shown="True" w392 {
          selector: w392 -> [_ w401]
          tunnel: w389 -> [w395 w398]
          tunnel: [w395 w397] -> w388
          tunnel: w391 -> [_ w400]
          frame False {
          }
          frame True {
            n169 = Not(x=w401) -> (.not. x?=w396:bool)
            n170 = call "Joystick.vi"("Joystick"=w396, "Gantry In"=w398) -> ("error out"=w399:errorcluster, "Gantry Out"=w397:refnum<k24>)  [unwired: 8 in]
            n171 = property class="Bool (strict)"(reference=w400, error in=w399, "Value"=w396) -> ()  [unwired: 2 out]
          }
        }
        n172 = call "ClearXYZTheta Go.vi"("Speed"=300.0, "XYZTheta In"=w394, "Gantry In"=w388) -> ("Gantry Out"=w387:refnum<k24>)  [unwired: 6 in, 2 out]
      }
      event "Go to Sensor ID": Value Change {
        n173 = event-data() -> ()  [unwired: 1 in, 6 out]
        n174 = Unbundle By Name(w409) -> ("Sensor ID Location"=w410:dbl[])
        n175 = control-ref of="Joystick"() -> (w406:refnum<vi>)
        n176 = property class="Bool (strict)"(reference=w406) -> (reference out=w407:refnum<vi>, "Value"=w408:bool)  [unwired: 1 in, 1 out]
        n177 = case shown="True" w408 {
          selector: w408 -> [_ w417]
          tunnel: w405 -> [w411 w414]
          tunnel: [w411 w413] -> w404
          tunnel: w407 -> [_ w416]
          frame False {
          }
          frame True {
            n178 = Not(x=w417) -> (.not. x?=w412:bool)
            n179 = call "Joystick.vi"("Joystick"=w412, "Gantry In"=w414) -> ("error out"=w415:errorcluster, "Gantry Out"=w413:refnum<k24>)  [unwired: 8 in]
            n180 = property class="Bool (strict)"(reference=w416, error in=w415, "Value"=w412) -> ()  [unwired: 2 out]
          }
        }
        n181 = call "ClearXYZTheta Go.vi"("Speed"=300.0, "XYZTheta In"=w410, "Gantry In"=w404) -> ("Gantry Out"=w403:refnum<k24>)  [unwired: 6 in, 2 out]
      }
      event "Verify CH1": Value Change {
        n182 = event-data() -> ()  [unwired: 1 in, 6 out]
        "CH1 correct?" <- TRUE
      }
    }
  }
  "Gantry Out" <- w7
